vi "write trace to 2D array.vi"(6 "Input array":dbl[](array[numeric]), 7 "Number of points":i32=601, 8 "error in (no error)":errorcluster, 9 "Linear Increment (MHz)":dbl=0.449251 format="%#_13g", 10 "Start F (MHz)":dbl=30.0 format="%#_13g", 11 "Visa in":refnum<visa-resource-name>) -> (0 "error out":errorcluster, 1 "Frequency VS Amplitude (2D array)":dbl[][](array[numeric]), 2 "Frequency in MHz (1D array)":dbl[](array[numeric]), 3 "VISA resource name":refnum<visa-resource-name>, 5 "size(s)":i32)   [LabVIEW 2016]
doc: "Write a trace (using t0, dt, Y-1D Array information) into CSV file, a 2D Array will be generated and saved in CSV file recording frequency VS amplitude."
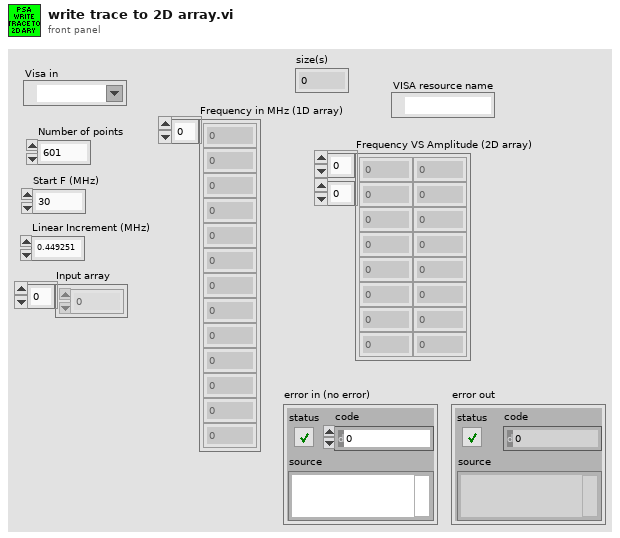
[diagram p1: front panel]
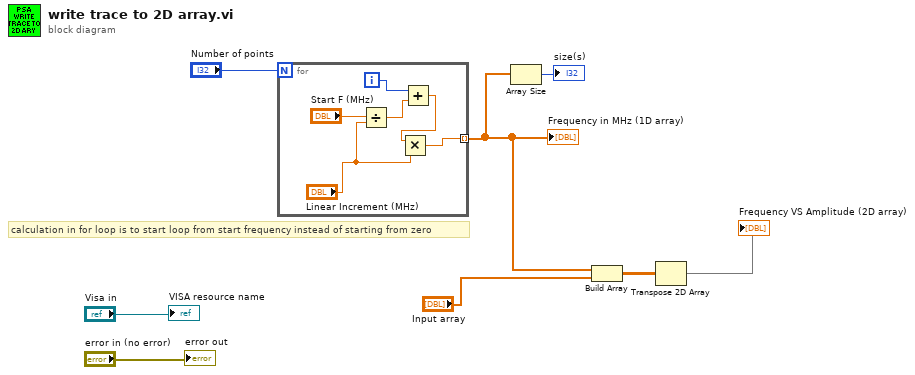
[diagram p0: block diagram]
diagram:
  # "calculation in for loop is to start loop from start frequency instead of starting from zero"
  n1 = for {
    N: "Number of points" -> [_]
    tunnel: [w14] -> w6 mode=indexing
    i -> [w13]
    n2 = Divide(x="Start F (MHz)", y="Linear Increment (MHz)") -> (x/y=w10:dbl)
    n3 = Add(x=w13, y=w10) -> (x+y=w9:dbl)
    n4 = Multiply(x=w9, y="Linear Increment (MHz)") -> (x*y=w14:dbl)
  }
  "Frequency in MHz (1D array)" <- w6
  n5 = Array Size(array=w6) -> (size(s)=→"size(s)":i32)
  n6 = Build Array(w6, "Input array") -> (w4:dbl[][])
  n7 = Transpose 2D Array(2D array=w4) -> (transposed array=→"Frequency VS Amplitude (2D array)":dbl[][])
  "error out" <- "error in (no error)"
  "VISA resource name" <- "Visa in"
